vi "Continuous_Measurement_v2.vi"() -> ()   [LabVIEW 2014]
uses:
  <vilib>/Analysis/NI_AALBase.lvlib
panel:
  out "V-I Graph 2":cluster{dbl[], dbl[]}(graph)
  out "I-t Graph 2":cluster{dbl[], dbl[]}(graph)
  out "V-t Graph 2":cluster{dbl[], dbl[]}(graph)
  out "TIV":dbl[][](array[numeric])
  in  "stop":bool
  out "I-t Graph":cluster{dbl[], dbl[]}(graph)
  out "V-t Graph":cluster{dbl[], dbl[]}(graph)
  out "V-I Graph":cluster{dbl[], dbl[]}(graph)
  out "Current Path":path
  in  "Meas. wait time (ms)":i32
  in  "Meas. to Avg":i32
  out "Voltage (V)":string
  in  "Current (uA)":dbl
  in  "Collect":bool
  in  "Outp. wait time (ms)":i32
  in  "2182A VISA":refnum<visa-resource-name>
  in  "Output Response":bool
  in  "Compliance (V)":dbl
  out "File Counter":i32
  out "Data Counter":i32
  in  "6221 VISA":refnum<visa-resource-name>
  in  "First Path":path
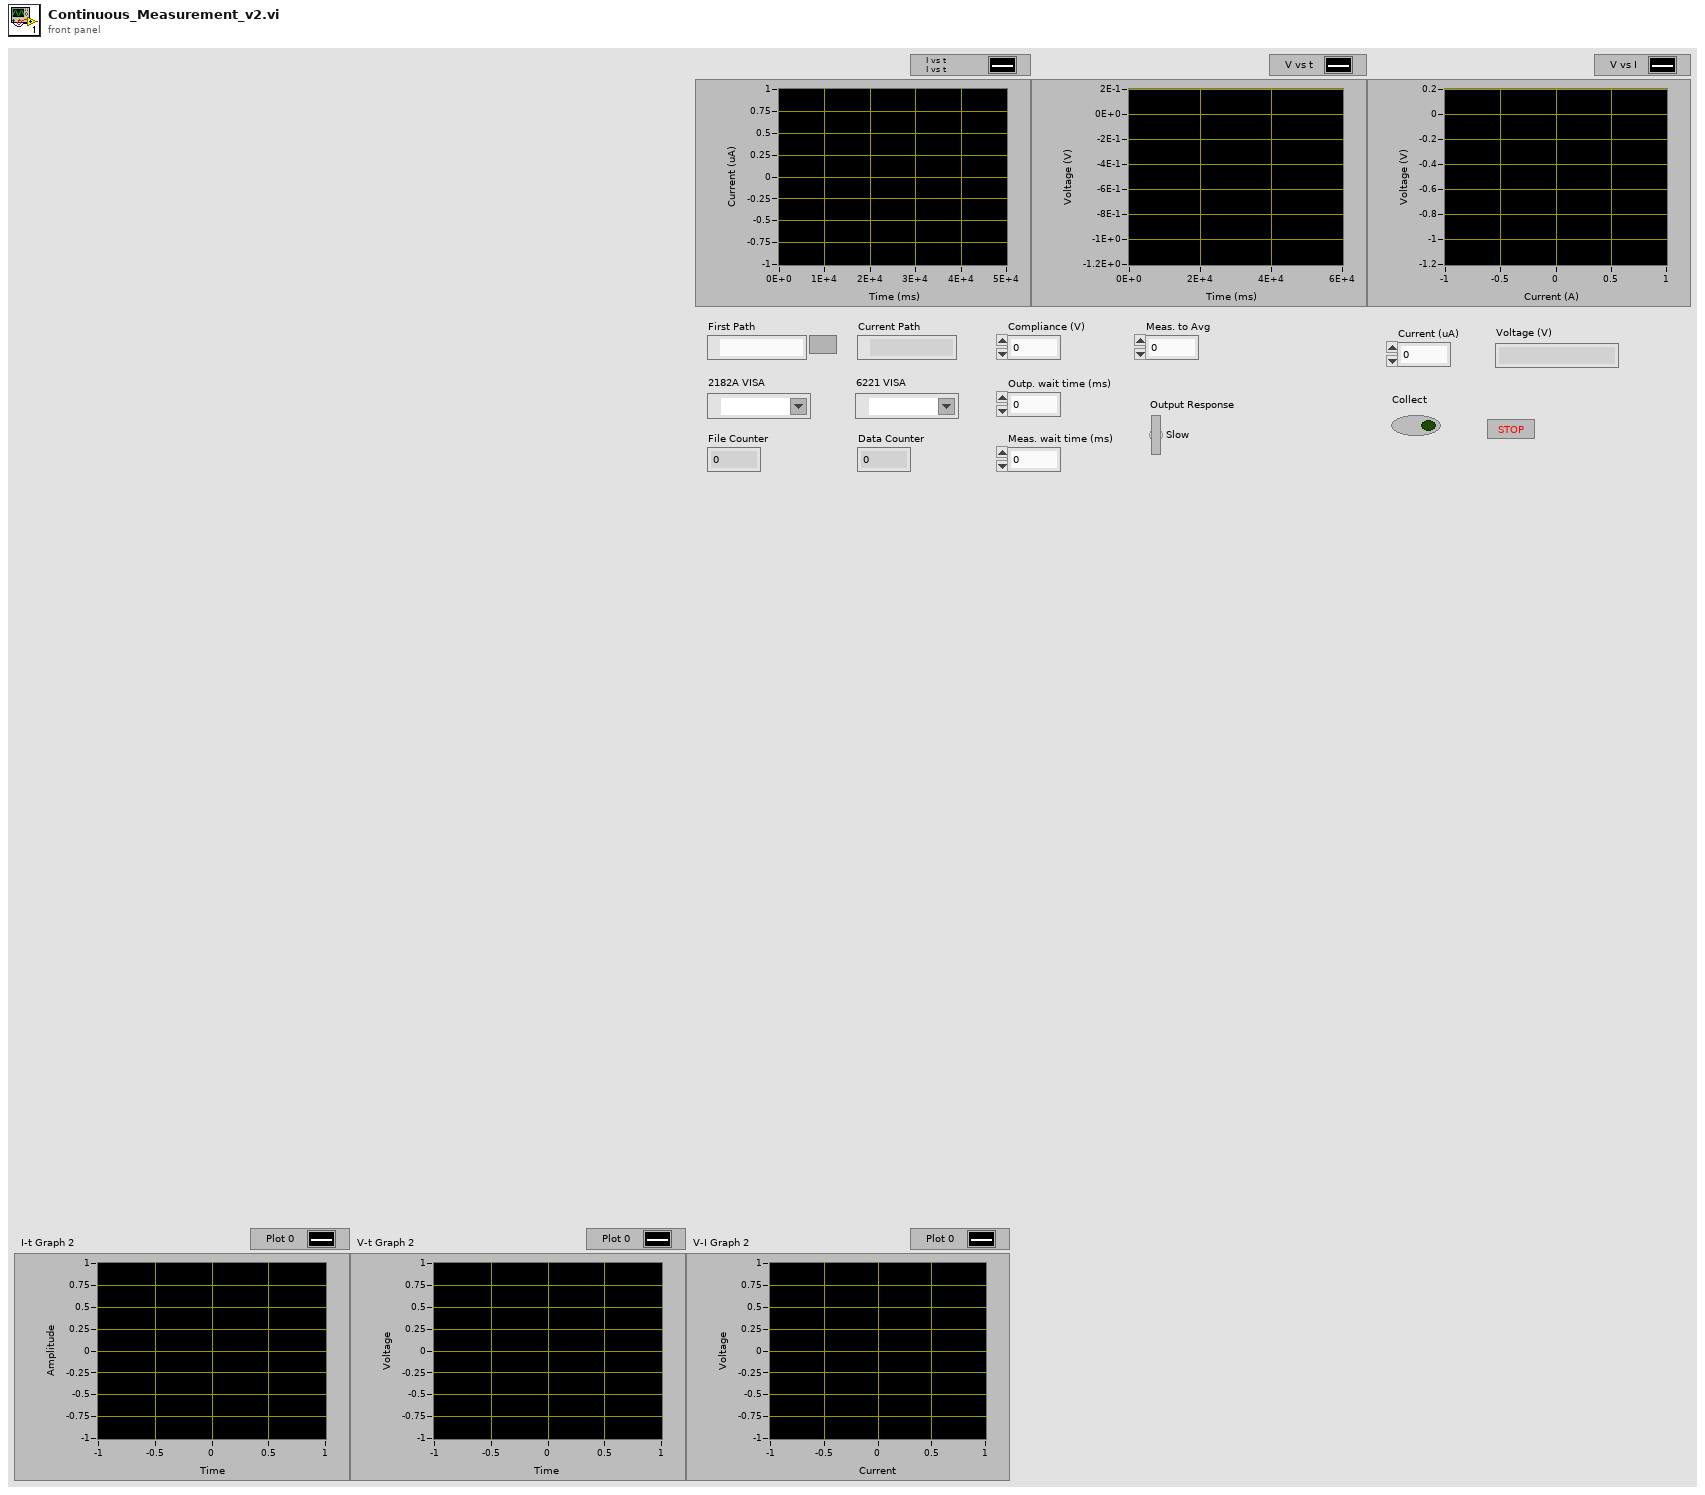
[diagram p1: front panel]
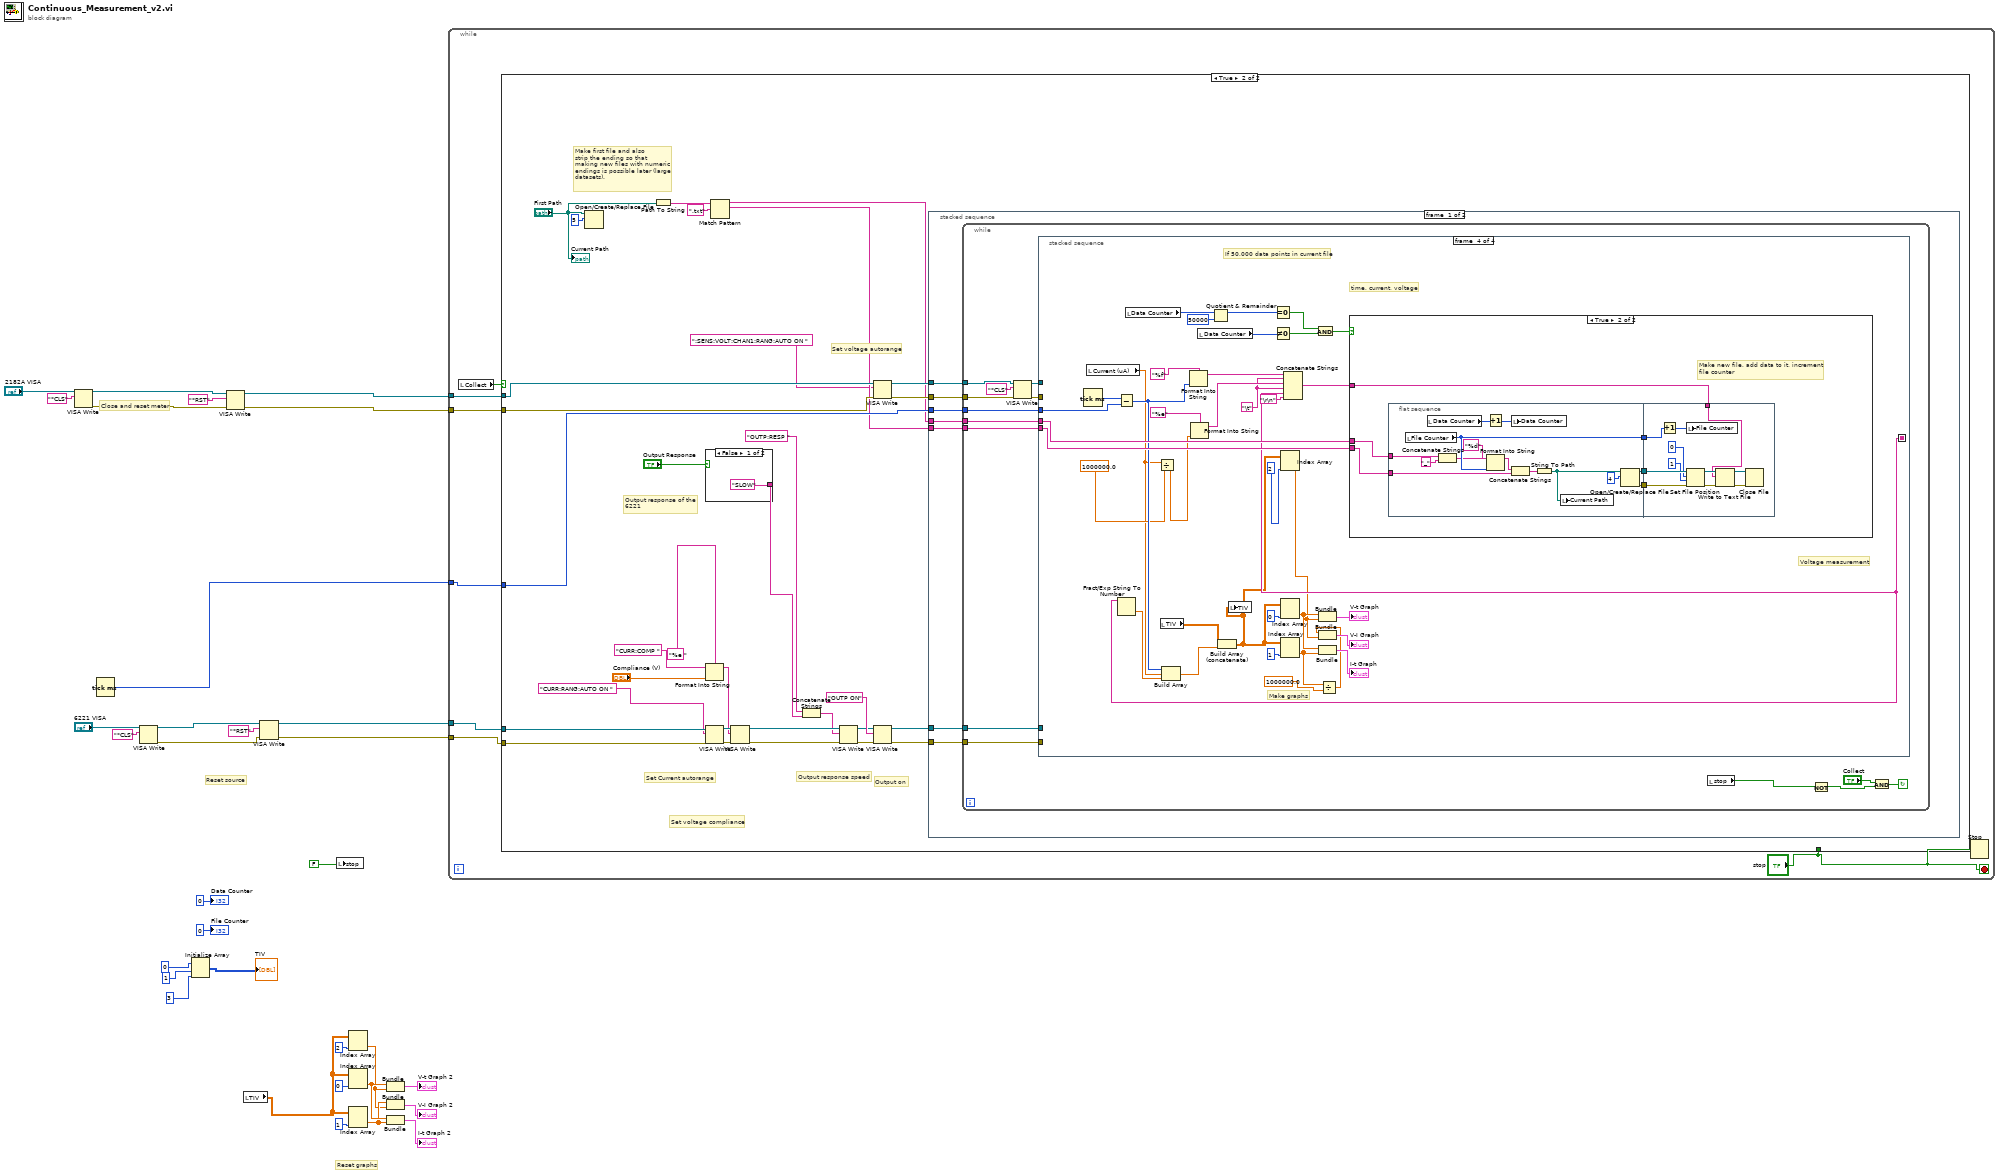
[diagram p0: block diagram]
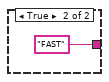
[diagram p3: hidden frame]
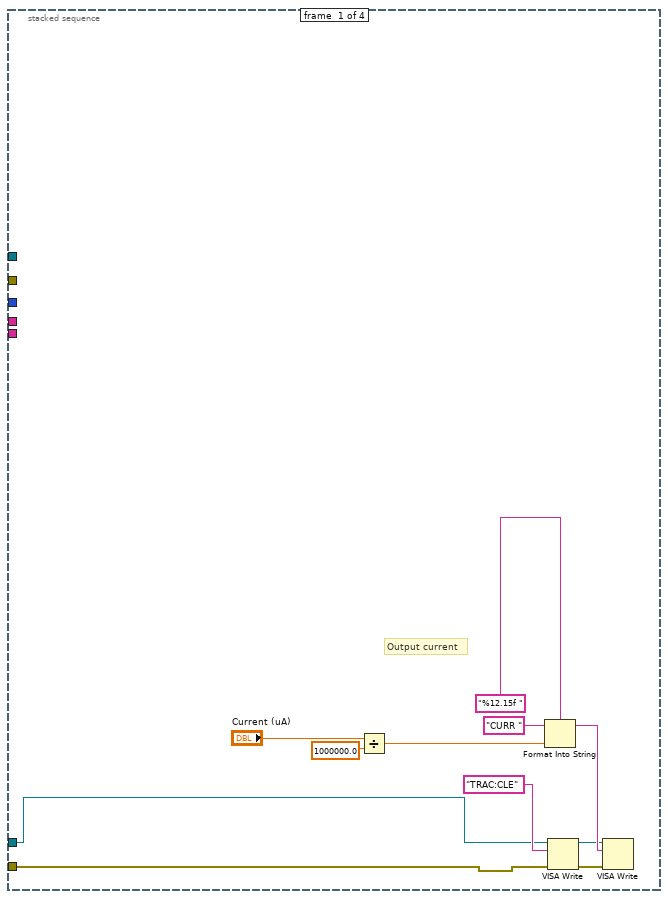
[diagram p4: hidden frame]
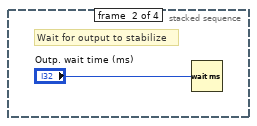
[diagram p5: hidden frame]
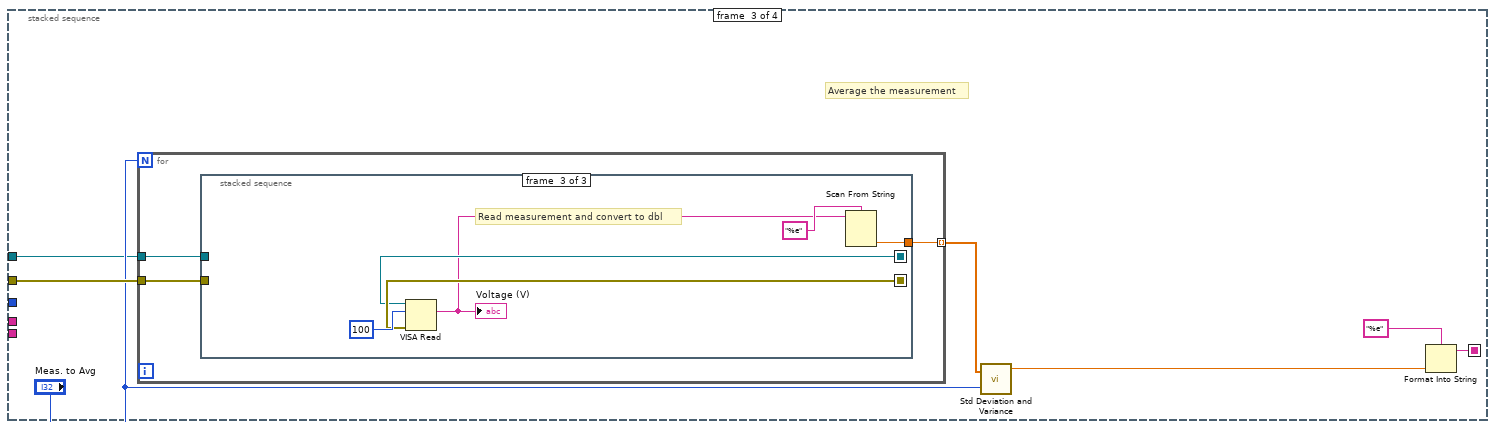
[diagram p6: hidden frame]
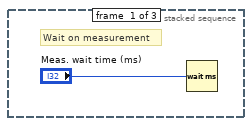
[diagram p7: hidden frame]
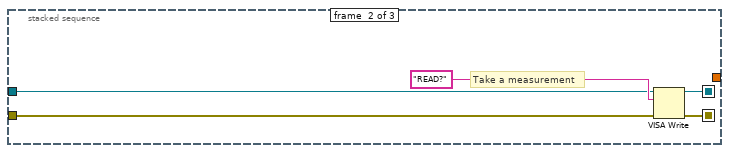
[diagram p8: hidden frame]
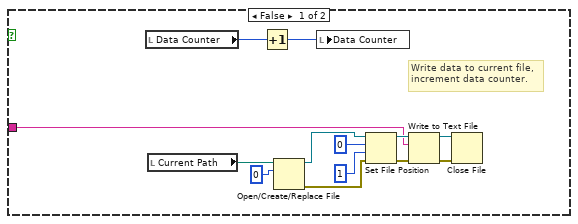
[diagram p9: hidden frame]
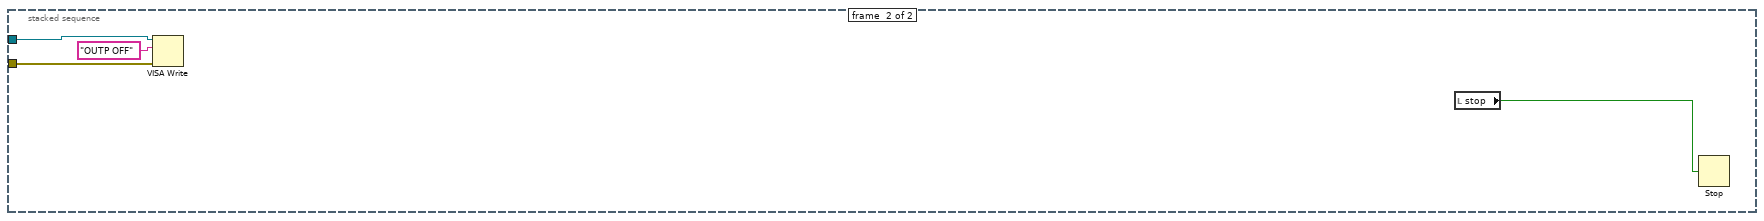
[diagram p10: hidden frame]
diagram:
  # "Reset graphs"
  # "Reset source"
  # "Close and reset meter"
  n1 = VISA Write(VISA resource name="2182A VISA", write buffer="*CLS") -> (VISA resource name out=w24:refnum<visa-resource-name>, error out=w29:errorcluster)  [unwired: 1 in, 1 out]
  n2 = Tick Count (ms)() -> (millisecond timer value=w16:u32)
  n3 = VISA Write(VISA resource name="6221 VISA", write buffer="*CLS") -> (VISA resource name out=w17:refnum<visa-resource-name>, error out=w18:errorcluster)  [unwired: 1 in, 1 out]
  n4 = Initialize Array(0, 1, 3) -> (→"TIV":i32[][])
  n5 = VISA Write(VISA resource name=w24, write buffer="*RST", error in (no error)=w29) -> (VISA resource name out=w23:refnum<visa-resource-name>, error out=w22:errorcluster)  [unwired: 1 out]
  n6 = local read "TIV"() -> (w1:dbl[][])
  n7 = VISA Write(VISA resource name=w17, write buffer="*RST", error in (no error)=w18) -> (VISA resource name out=w20:refnum<visa-resource-name>, error out=w19:errorcluster)  [unwired: 1 out]
  n8 = local write "stop"(FALSE) -> ()
  n9 = Index Array(array=w1, index (col)=2) -> (element=w3:dbl[])  [unwired: 1 in]
  n10 = Index Array(array=w1, index (col)=0) -> (element=w6:dbl[])  [unwired: 1 in]
  n11 = Index Array(array=w1, index (col)=1) -> (element=w4:dbl[])  [unwired: 1 in]
  n12 = Bundle("TIV"=w6, "TIV"=w3) -> (→"V-t Graph 2":cluster{"TIV":dbl[], "TIV":dbl[]})  [unwired: 1 in]
  n13 = Bundle("TIV"=w4, "TIV"=w3) -> (→"V-I Graph 2":cluster{"TIV":dbl[], "TIV":dbl[]})  [unwired: 1 in]
  n14 = Bundle("TIV"=w6, "TIV"=w4) -> (→"I-t Graph 2":cluster{"TIV":dbl[], "TIV":dbl[]})  [unwired: 1 in]
  n15 = while {
    tunnel: w23 -> [w38]
    tunnel: w22 -> [w37]
    tunnel: w20 -> [w36]
    tunnel: w19 -> [w35]
    tunnel: w16 -> [w34]
    stop <- "stop" stop-if-true
    n16 = local read "Collect"() -> (w39:bool)
    n17 = case shown="True" w39 {
      tunnel: w37 -> [_ w51]
      tunnel: w38 -> [_ w52]
      tunnel: w36 -> [_ w50]
      tunnel: w35 -> [_ w49]
      tunnel: w34 -> [_ w48]
      tunnel: "stop" -> [_ _]
      frame False {
      }
      frame True {
        # "Output on"
        # "Output response of the\n6221"
        # "Make first file and also\nstrip the ending so that\nmaking new files with numeric\nendings is possible later (large\ndatasets)."
        # "Output response speed"
        # "Set voltage compliance"
        # "Set Current autorange"
        # "Set voltage autorange"
        n18 = Open/Create/Replace File(file path (use dialog)="First Path", operation (0:open)=5) -> ()  [unwired: 4 in, 3 out]
        n19 = Path To String(path="First Path") -> (string=w46:string)
        n20 = case shown="False" "Output Response" {
          tunnel: ["SLOW" "FAST"] -> w62
          frame False {
          }
          frame True {
          }
        }
        n21 = Format Into String(format string="%e ", initial string="CURR:COMP ", "Compliance (V)") -> (resulting string=w60:string)  [unwired: 1 in, 1 out]
        n22 = VISA Write(VISA resource name=w50, write buffer="CURR:RANG:AUTO ON ", error in (no error)=w49) -> (VISA resource name out=w65:refnum<visa-resource-name>, error out=w66:errorcluster)  [unwired: 1 out]
        n23 = Match Pattern(string=w46, regular expression=".txt") -> (before substring=w43:string, match substring=w42:string)  [unwired: 1 in, 2 out]
        n24 = VISA Write(VISA resource name=w65, write buffer=w60, error in (no error)=w66) -> (VISA resource name out=w68:refnum<visa-resource-name>, error out=w67:errorcluster)  [unwired: 1 out]
        n25 = Concatenate Strings("OUTP:RESP ", w62) -> (w64:string)
        n26 = VISA Write(VISA resource name=w68, write buffer=w64, error in (no error)=w67) -> (VISA resource name out=w56:refnum<visa-resource-name>, error out=w55:errorcluster)  [unwired: 1 out]
        n27 = VISA Write(VISA resource name=w52, write buffer=":SENS:VOLT:CHAN1:RANG:AUTO ON ", error in (no error)=w51) -> (VISA resource name out=w54:refnum<visa-resource-name>, error out=w53:errorcluster)  [unwired: 1 out]
        n28 = VISA Write(VISA resource name=w56, write buffer="OUTP ON", error in (no error)=w55) -> (VISA resource name out=w70:refnum<visa-resource-name>, error out=w69:errorcluster)  [unwired: 1 out]
        n29 = stacked-sequence {
          tunnel: w69 -> [w80 w214]
          tunnel: w53 -> [w79 _]
          tunnel: w48 -> [w78 _]
          tunnel: w43 -> [w77 _]
          tunnel: w42 -> [w76 _]
          tunnel: w70 -> [w75 w212]
          tunnel: w54 -> [w74 _]
          frame #0 {
            n30 = while {
              tunnel: w80 -> [w94]
              tunnel: w79 -> [w92]
              tunnel: w78 -> [w90]
              tunnel: w77 -> [w89]
              tunnel: w76 -> [w88]
              tunnel: w75 -> [w84]
              tunnel: w74 -> [w83]
              stop <- w85 continue-if-true
              n31 = VISA Write(VISA resource name=w83, write buffer="*CLS", error in (no error)=w92) -> (VISA resource name out=w82:refnum<visa-resource-name>, error out=w91:errorcluster)  [unwired: 1 out]
              n32 = stacked-sequence {
                seq-local: [_ _ w109 _] -> [_ _ _ w146]
                tunnel: w94 -> [w95 _ _ _]
                tunnel: w91 -> [_ _ w113 _]
                tunnel: w90 -> [_ _ _ w165]
                tunnel: w89 -> [_ _ _ w152]
                tunnel: w88 -> [_ _ _ w151]
                tunnel: w84 -> [w96 _ _ _]
                tunnel: w82 -> [_ _ w108 _]
                frame #0 {
                  # "Output current"
                  n33 = Divide(x="Current (uA)", y=1000000.0) -> (x/y=w98:dbl)
                  n34 = Format Into String(format string="%12.15f ", initial string="CURR ", w98) -> (resulting string=w101:string)  [unwired: 1 in, 1 out]
                  n35 = VISA Write(VISA resource name=w96, write buffer="TRAC:CLE", error in (no error)=w95) -> (VISA resource name out=w97:refnum<visa-resource-name>, error out=w104:errorcluster)  [unwired: 1 out]
                  n36 = VISA Write(VISA resource name=w97, write buffer=w101, error in (no error)=w104) -> ()  [unwired: 3 out]
                }
                frame #1 {
                  # "Wait for output to stabilize"
                  n37 = Wait (ms)(milliseconds to wait="Outp. wait time (ms)") -> ()  [unwired: 1 out]
                }
                frame #2 {
                  # "Average the measurement"
                  n38 = for {
                    N: "Meas. to Avg" -> [_]
                    tunnel: w113 -> [w116]
                    tunnel: [w115] -> w112 mode=indexing
                    tunnel: w108 -> [w114]
                    n39 = stacked-sequence {
                      seq-local: [_ w120 _] -> [_ _ w127]
                      seq-local: [_ w118 _] -> [_ _ w124]
                      tunnel: w116 -> [_ w121 _]
                      tunnel: [_ _ w125] -> w115
                      tunnel: w114 -> [_ w119 _]
                      frame #0 {
                        # "Wait on measurement"
                        n40 = Wait (ms)(milliseconds to wait="Meas. wait time (ms)") -> ()  [unwired: 1 out]
                      }
                      frame #1 {
                        # "Take a measurement"
                        n41 = VISA Write(VISA resource name=w119, write buffer="READ?", error in (no error)=w121) -> (VISA resource name out=w118:refnum<visa-resource-name>, error out=w120:errorcluster)  [unwired: 1 out]
                      }
                      frame #2 {
                        # "Read measurement and convert to dbl"
                        n42 = VISA Read(VISA resource name=w124, byte count=100, error in (no error)=w127) -> (read buffer=w123:string)  [unwired: 3 out]
                        "Voltage (V)" <- w123
                        n43 = Scan From String(format string="%e", input string=w123) -> (output 1=w125:dbl)  [unwired: 3 in, 3 out]
                      }
                    }
                  }
                  n44 = call <vilib>:"Std Deviation and Variance.vi"("X"=w112, "Weighting (Sample)"="Meas. to Avg") -> ("mean"=w107:dbl)  [unwired: 2 out]
                  n45 = Format Into String(format string="%e", w107) -> (resulting string=w109:string)  [unwired: 2 in, 1 out]
                }
                frame #3 {
                  w160 = "\t"
                  # "Make graphs"
                  # "time, current, voltage"
                  # "If 50,000 data points in current file"
                  # "Voltage measurement"
                  n46 = Tick Count (ms)() -> (millisecond timer value=w166:u32)
                  n47 = local read "Current (uA)"() -> (w133:dbl)
                  n48 = Fract/Exp String To Number(string=w146) -> (number=w145:dbl)  [unwired: 3 in, 1 out]
                  n49 = Subtract(x=w166, y=w165) -> (x-y=w148:u32)
                  n50 = local read "Data Counter"() -> (w158:i32)
                  n51 = Divide(x=w133, y=1000000.0) -> (x/y=w135:dbl)
                  n52 = local read "TIV"() -> (w149:dbl[][])
                  n53 = Build Array(w148, w133, w145) -> (w147:dbl[])
                  n54 = Format Into String(format string="%f", w148) -> (resulting string=w163:string)  [unwired: 2 in, 1 out]
                  n55 = Format Into String(format string="%e", w135) -> (resulting string=w161:string)  [unwired: 2 in, 1 out]
                  n56 = local read "Data Counter"() -> (w155:i32)
                  n57 = Quotient & Remainder(x=w158, y=50000) -> (x-y*floor(x/y)=w129:i32)  [unwired: 1 out]
                  n58 = Build Array (concatenate)(w149, w147) -> (w136:dbl[][])
                  n59 = local write "TIV"(w136) -> ()
                  n60 = Equal To 0?(x=w129) -> (x = 0?=w156:bool)
                  n61 = Not Equal To 0?(x=w155) -> (x != 0?=w154:bool)
                  n62 = Index Array(array=w136, index (col)=2) -> (element=w138:dbl[])  [unwired: 1 in]
                  n63 = Index Array(array=w136, index (col)=0) -> (element=w140:dbl[])  [unwired: 1 in]
                  n64 = Index Array(array=w136, index (col)=1) -> (element=w132:dbl[])  [unwired: 1 in]
                  n65 = Concatenate Strings(w163, w160, w161, w160, w146, "\r\n") -> (w150:string)
                  n66 = And(x=w156, y=w154) -> (x .and. y?=w153:bool)
                  n67 = Bundle(w140, w138) -> (→"V-t Graph":cluster{dbl[], dbl[]})  [unwired: 1 in]
                  n68 = Bundle(w140, w132) -> (→"I-t Graph":cluster{dbl[], dbl[]})  [unwired: 1 in]
                  n69 = Divide(x=w132, y=1000000.0) -> (x/y=w130:dbl[])
                  n70 = Bundle(w130, w138) -> (→"V-I Graph":cluster{dbl[], dbl[]})  [unwired: 1 in]
                  n71 = case shown="True" w153 {
                    tunnel: w152 -> [_ w184]
                    tunnel: w151 -> [_ w183]
                    tunnel: w150 -> [w173 w181]
                    frame False {
                      # "Write data to current file,\nincrement data counter."
                      n72 = local read "Data Counter"() -> (w172:i32)
                      n73 = local read "Current Path"() -> (w179:path)
                      n74 = Increment(x=w172) -> (x+1=w171:i32)
                      n75 = Open/Create/Replace File(file path (use dialog)=w179, operation (0:open)=0) -> (refnum out=w177:refnum<file>, error out=w167:errorcluster)  [unwired: 4 in, 1 out]
                      n76 = local write "Data Counter"(w171) -> ()
                      n77 = Set File Position(offset (in bytes) (0)=0, refnum=w177, from (0:start)=1, error in=w167) -> (refnum out=w174:refnum<file>, error out=w168:errorcluster)
                      n78 = Write to Text File(file (use dialog)=w174, text=w173, error in=w168) -> (refnum out=w169:refnum<file>, error out=w170:errorcluster)  [unwired: 1 in, 1 out]
                      n79 = Close File(refnum=w169, error in=w170) -> ()  [unwired: 2 out]
                    }
                    frame True {
                      # "Make new file, add data to it, increment\nfile counter"
                      n80 = flat-sequence {
                        tunnel: [w199] -> w185
                        tunnel: w184 -> [w197]
                        tunnel: w183 -> [w192]
                        tunnel: [w189] -> w182
                        tunnel: [w188] -> w180
                        tunnel: w185 -> [w210]
                        tunnel: w182 -> [w208]
                        tunnel: w181 -> [w204]
                        tunnel: w180 -> [w202]
                        frame #0 {
                          n81 = local read "File Counter"() -> (w199:i32)
                          n82 = local read "Data Counter"() -> (w187:i32)
                          n83 = Concatenate Strings(w197, "_") -> (w196:string)
                          n84 = Format Into String(format string="%d", initial string=w196, w199) -> (resulting string=w193:string)  [unwired: 1 in, 1 out]
                          n85 = Increment(x=w187) -> (x+1=w186:i32)
                          n86 = local write "Data Counter"(w186) -> ()
                          n87 = Concatenate Strings(w193, w192) -> (w194:string)
                          n88 = String To Path(string=w194) -> (path=w190:path)
                          n89 = local write "Current Path"(w190) -> ()
                          n90 = Open/Create/Replace File(file path (use dialog)=w190, operation (0:open)=4) -> (refnum out=w189:refnum<file>, error out=w188:errorcluster)  [unwired: 4 in, 1 out]
                        }
                        frame #1 {
                          n91 = Increment(x=w210) -> (x+1=w209:i32)
                          n92 = local write "File Counter"(w209) -> ()
                          n93 = Set File Position(offset (in bytes) (0)=0, refnum=w208, from (0:start)=1, error in=w202) -> (refnum out=w205:refnum<file>, error out=w203:errorcluster)
                          n94 = Write to Text File(file (use dialog)=w205, text=w204, error in=w203) -> (refnum out=w200:refnum<file>, error out=w201:errorcluster)  [unwired: 1 in, 1 out]
                          n95 = Close File(refnum=w200, error in=w201) -> ()  [unwired: 2 out]
                        }
                      }
                    }
                  }
                }
              }
              n96 = local read "stop"() -> (w81:bool)
              n97 = Not(x=w81) -> (.not. x?=w86:bool)
              n98 = And(x="Collect", y=w86) -> (x .and. y?=w85:bool)
            }
          }
          frame #1 {
            n99 = VISA Write(VISA resource name=w212, write buffer="OUTP OFF", error in (no error)=w214) -> ()  [unwired: 3 out]
            n100 = local read "stop"() -> (w211:bool)
            n101 = Stop(stop? (T)=w211) -> ()
          }
        }
        "Current Path" <- "First Path"
      }
    }
    n102 = Stop(stop? (T)="stop") -> ()
  }
  "Data Counter" <- 0
  "File Counter" <- 0
